vi "data Cluster.vi"(11 "Data Array":dbl[](array[numeric])) -> (3 "Data Cluster":T1)   [LabVIEW 2021, in "IMU Processing.lvlib"]
uses:
  IMU Processing.lvlib
  data.ctl
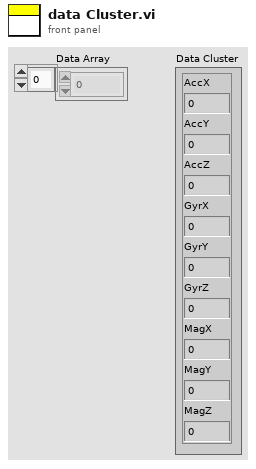
[diagram p1: front panel]
types:
  T1 = typedef "IMU Processing.lvlib/data.ctl" = cluster{"AccX":dbl, "AccY":dbl, "AccZ":dbl, "GyrX":dbl, "GyrY":dbl, "GyrZ":dbl, "MagX":dbl, "MagY":dbl, "MagZ":dbl}
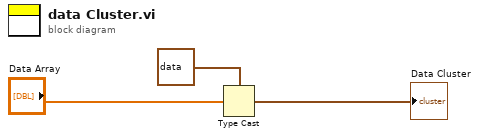
[diagram p0: block diagram]
diagram:
  n1 = Type Cast(type=T1 {"AccX"=0.0, "AccY"=0.0, "AccZ"=0.0, "GyrX"=0.0, "GyrY"=0.0, "GyrZ"=0.0, "MagX"=0.0, "MagY"=0.0, "MagZ"=0.0}, x="Data Array") -> (*(type *) &x=→"Data Cluster":T1)
